vi "ClsInit.vi"(8 "error in (no error)":errorcluster, 11 "ClsInit 2":T1) -> (0 "error out":errorcluster, 3 "Connection Out out":u32)   [LabVIEW 2015]
uses:
  TypeDefs/ClsSettings.ctl
  ClsSendCmds_Array.vi
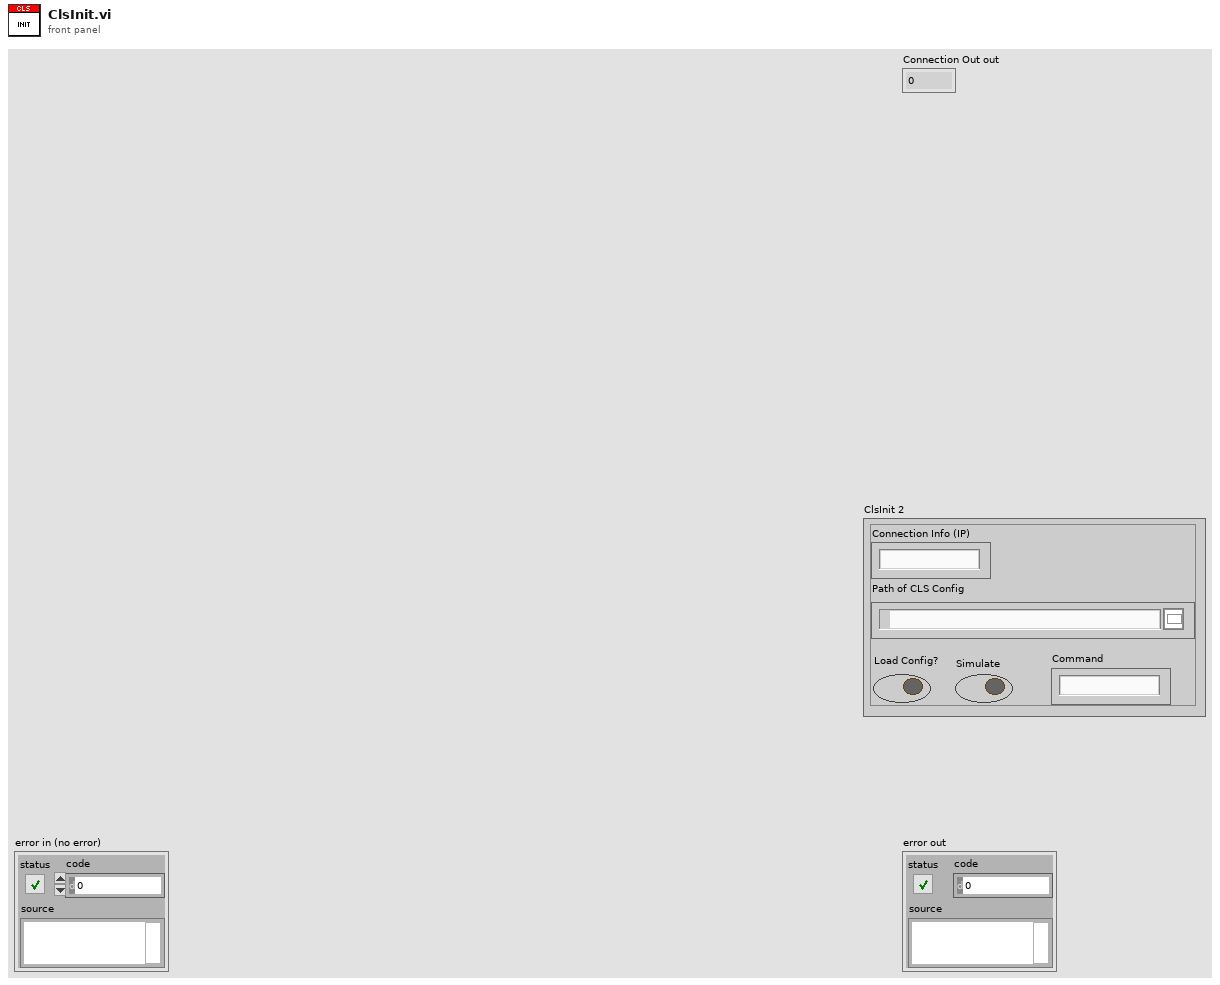
[diagram p1: front panel]
types:
  T1 = typedef "ClsSettings.ctl" = cluster{"Connection Info (IP)":string, "Simulate":bool, "Load Config?":bool, "Path of CLS Config":path, "Command ":string}
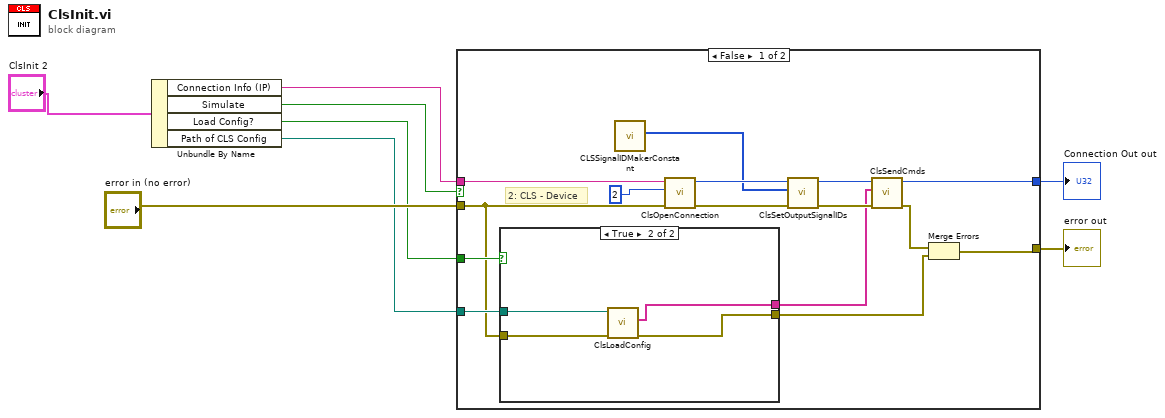
[diagram p0: block diagram]
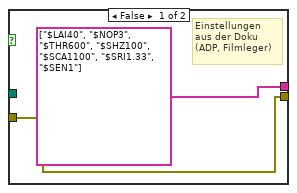
[diagram p2: hidden frame]
diagram:
  n1 = Unbundle By Name("ClsInit 2") -> ("Connection Info (IP)"=w4:string, "Simulate"=w3:bool, "Load Config?"=w2:bool, "Path of CLS Config"=w1:path)
  n2 = case shown="False" w3 {
    tunnel: "error in (no error)" -> [w12 w30]
    tunnel: w4 -> [w23 _]
    tunnel: [w9 w30] -> w8
    tunnel: w2 -> [w19 _]
    tunnel: [w16 _] -> w6
    tunnel: w1 -> [w13 _]
    frame False {
      # "2: CLS - Device"
      n3 = case shown="True" w19 {
        tunnel: [string[] ["$LAI40", "$NOP3", "$THR600", "$SHZ100", "$SCA1100", "$SRI1.33", "$SEN1"] ("InitCommandArray") w28] -> w15
        tunnel: w13 -> [_ w29]
        tunnel: w12 -> [w24 w27]
        tunnel: [w24 w26] -> w10
        frame False {
          # "Einstellungen\naus der Doku\n(ADP, Filmleger)"
        }
        frame True {
          n4 = call "ClsLoadConfig.vi"("error in (no error)"=w27, "XML File Path"=w29) -> ("error out"=w26:errorcluster, "ClsCondigureValues (Array)"=w28:string[])  [unwired: 7 in, 1 out]
        }
      }
      n5 = call "CLSSignalIDMakerConstant.vi"() -> ("SignalID"=w14:i32[])  [unwired: 11 in]
      n6 = call "ClsOpenConnection.vi"("error in"=w12, "Device Type"=2, "Connection Info"=w23) -> ("error out"=w22:errorcluster, "Connection Handle out"=w21:u32)  [unwired: 5 in]
      n7 = call "ClsSetOutputSignalIDs.vi"("error in (no error)"=w22, "Signal IDs array"=w14, "Connection In"=w21) -> ("error out"=w17:errorcluster, "Connection Out"=w18:u32)  [unwired: 7 in]
      n8 = call-poly "ClsSendCmds.vi"("error in (no error)"=w17, "InitCommandArray"=w15, "Connection Out in"=w18) -> ("error out"=w11:errorcluster, "Connection Out out"=w16:u32)  [unwired: 6 in, 1 out]
      n9 = Merge Errors(w11, w10) -> (w9:errorcluster)
    }
    frame True {
    }
  }
  "error out" <- w8
  "Connection Out out" <- w6
